vi "Read GroupName.vi"(8 "error in":errorcluster, 11 "group in":refnum<class "group node.lvclass">) -> (0 "error out":errorcluster, 2 "groupName":string, 3 "group out":refnum<class "group node.lvclass">)   [LabVIEW 2013, in "group node.lvclass"]
uses:
  group node.lvclass
  group node.lvclass/group node.ctl
  CEF_TreeControl/serializable configuration/read metadata property.vi
  group configuration/group configuration.lvclass
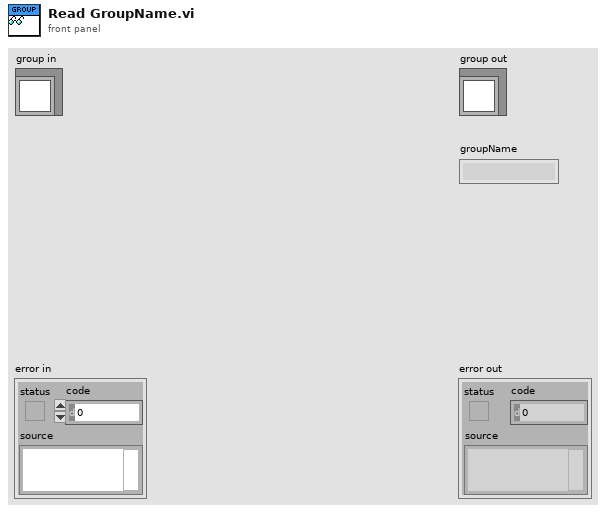
[diagram p1: front panel]
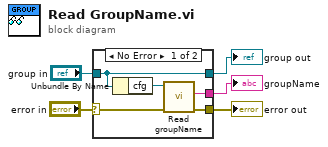
[diagram p0: block diagram]
diagram:
  n1 = case shown="No Error" "error in" {
    selector: "error in" -> [w8 w11]
    tunnel: [w7 w11] -> w4
    tunnel: [w10 w12] -> w2
    tunnel: "group in" -> [w10 w12]
    tunnel: [w6 _] -> w1
    frame No Error {
      n2 = Unbundle By Name(w10) -> ("cfg"=w9:refnum<class "group configuration.lvclass">)
      n3 = call "Read groupName.vi"("error in"=w8, "group configuration in"=w9) -> ("error out"=w7:errorcluster, "groupName"=w6:string)  [unwired: 7 in, 1 out]
    }
    frame Error {
    }
  }
  "error out" <- w4
  "group out" <- w2
  "groupName" <- w1
